vi "Format CSV.vi"(8 "error in (no error)":errorcluster, 9 "delimiter":string=",", 10 "CSV File Input":path, 11 "Original CSV Format":enum16{"Format A", "Format B"}(ring)) -> (0 "error out":errorcluster, 1 "Parcel Length":i32[](array[numeric]), 2 "All Terminal Data":T1(array[cluster]))   [LabVIEW 2017] (continued)
"46:50.6", "46:50.7", "46:50.7", "46:50.7", "46:50.8", "46:50.8", "46:50.8", "46:50.9", "46:50.9", "46:50.9", "46:51.0", "46:51.0", "46:51.0", "46:51.1", "46:51.1", "46:51.1", "46:51.2", "46:51.2", "46:51.2", "46:51.3", "46:51.3", "46:51.3", "46:51.4", "46:51.4", "46:51.4", "46:51.5", "46:51.5", "46:51.5", "46:51.6", "46:51.6", "46:51.6", "46:51.7", "46:51.7", "46:51.7", "46:51.8", "46:51.8", "46:51.8", "46:51.9", "46:51.9", "46:51.9", "46:52.0", "46:52.0", "46:52.0", "46:52.1", "46:52.1", "46:52.1", "46:52.2", "46:52.2", "46:52.2", "46:52.3", "46:52.3", "46:52.3", "46:52.4", "46:52.4", "46:52.4", "46:52.5", "46:52.5", "46:52.5", "46:52.6", "46:52.6", "46:52.6", "46:52.7", "46:52.7", "46:52.7", "46:52.8", "46:52.8", "46:52.8", "46:52.9", "46:52.9", "46:52.9", "46:53.0", "46:53.0", "46:53.0", "46:53.1", "46:53.1", "46:53.1", "46:53.2", "46:53.2", "46:53.2", "46:53.3", "46:53.3", "46:53.3", "46:53.4", "46:53.4", "46:53.4", "46:53.5", "46:53.5", "46:53.5", "46:53.6", "46:53.6", "46:53.6", "46:53.7", "46:53.7", "46:53.7", "46:53.8", "46:53.8", "46:53.8", "46:53.9", "46:53.9", "46:53.9", "46:54.0", "46:54.0", "46:54.0", "46:54.1", "46:54.1", "46:54.1", "46:54.2", "46:54.2", "46:54.2", "46:54.3", "46:54.3", "46:54.3", "46:54.4", "46:54.4", "46:54.4", "46:54.5", "46:54.5", "46:54.5", "46:54.6", "46:54.6", "46:54.6", "46:54.7", "46:54.7", "46:54.7", "46:54.8", "46:54.8", "46:54.8", "46:54.9", "46:54.9", "46:54.9", "46:55.0", "46:55.0", "46:55.0", "46:55.1", "46:55.1", "46:55.1", "46:55.2", "46:55.2", "46:55.2", "46:55.3", "46:55.3", "46:55.3", "46:55.4", "46:55.4", "46:55.4", "46:55.5", "46:55.5", "46:55.5", "46:55.6", "46:55.6", "46:55.6", "46:55.7", "46:55.7", "46:55.7", "46:55.8", "46:55.8", "46:55.8", "46:55.9", "46:55.9", "46:55.9", "46:56.0", "46:56.0", "46:56.0", "46:56.1", "46:56.1", "46:56.1", "46:56.2", "46:56.2", "46:56.2", "46:56.3", "46:56.3", "46:56.3", "46:56.4", "46:56.4", "46:56.4", "46:56.5", "46:56.5", "46:56.5", "46:56.6", "46:56.6", "46:56.6", "46:56.7", "46:56.7", "46:56.7", "46:56.8", "46:56.8", "46:56.8", "46:56.9", "46:56.9", "46:56.9", "46:57.0", "46:57.0", "46:57.0", "46:57.1", "46:57.1", "46:57.1", "46:57.2", "46:57.2", "46:57.2", "46:57.3", "46:57.3", "46:57.3", "46:57.4", "46:57.4", "46:57.4", "46:57.5", "46:57.5", "46:57.5", "46:57.6", "46:57.6", "46:57.6", "46:57.7", "46:57.7", "46:57.7", "46:57.8", "46:57.8", "46:57.8", "46:57.9", "46:57.9", "46:57.9", "46:58.0", "46:58.0", "46:58.0", "46:58.1", "46:58.1", "46:58.1", "46:58.2", "46:58.2", "46:58.2", "46:58.3", "46:58.3", "46:58.3", "46:58.4", "46:58.4", "46:58.4", "46:58.5", "46:58.5", "46:58.5", "46:58.6", "46:58.6", "46:58.6", "46:58.7", "46:58.7", "46:58.7", "46:58.8", "46:58.8", "46:58.8", "46:58.9", "46:58.9", "46:58.9", "46:59.0", "46:59.0", "46:59.0", "46:59.1", "46:59.1", "46:59.1", "46:59.2", "46:59.2", "46:59.2", "46:59.3", "46:59.3", "46:59.3", "46:59.4", "46:59.4", "46:59.4", "46:59.5", "46:59.5", "46:59.5", "46:59.6", "46:59.6", "46:59.6", "46:59.7", "46:59.7", "46:59.7", "46:59.8", "46:59.8", "46:59.8", "46:59.9", "46:59.9", "46:59.9", "47:00.0", "47:00.0", "47:00.0", "47:00.1", "47:00.1", "47:00.1", "47:00.2", "47:00.2", "47:00.2", "47:00.3", "47:00.3", "47:00.3", "47:00.4", "47:00.4", "47:00.4", "47:00.5", "47:00.5", "47:00.5", "47:00.6", "47:00.6", "47:00.6", "47:00.7", "47:00.7", "47:00.7", "47:00.8", "47:00.8", "47:00.8", "47:00.9", "47:00.9", "47:00.9", "47:01.0", "47:01.0", "47:01.0", "47:01.1", "47:01.1", "47:01.1", "47:01.2", "47:01.2", "47:01.2", "47:01.3", "47:01.3", "47:01.3", "47:01.4", "47:01.4", "47:01.4", "47:01.5", "47:01.5", "47:01.5", "47:01.6", "47:01.6", "47:01.6", "47:01.7", "47:01.7", "47:01.7", "47:01.8", "47:01.8", "47:01.8", "47:01.9", "47:01.9", "47:01.9", "47:02.0", "47:02.0", "47:02.0", "47:02.1", "47:02.1", "47:02.1", "47:02.2", "47:02.2", "47:02.2", "47:02.3", "47:02.3", "47:02.3", "47:02.4", "47:02.4", "47:02.4", "47:02.5", "47:02.5", "47:02.5", "47:02.6", "47:02.6", "47:02.6", "47:02.7", "47:02.7", "47:02.7", "47:02.8", "47:02.8", "47:02.8", "47:02.9", "47:02.9", "47:02.9", "47:03.0", "47:03.0", "47:03.0", "47:03.1", "47:03.1", "47:03.1", "47:03.2", "47:03.2", "47:03.2", "47:03.3", "47:03.3", "47:03.3", "47:03.4", "47:03.4", "47:03.4", "47:03.5", "47:03.5", "47:03.5", "47:03.6", "47:03.6", "47:03.6", "47:03.7", "47:03.7", "47:03.7", "47:03.8", "47:03.8", "47:03.8", "47:03.9", "47:03.9", "47:03.9", "47:04.0", "47:04.0", "47:04.0", "47:04.1", "47:04.1", "47:04.1", "47:04.2", "47:04.2", "47:04.2", "47:04.3", "47:04.3", "47:04.3", "47:04.4", "47:04.4", "47:04.4", "47:04.5", "47:04.5", "47:04.5", "47:04.6", "47:04.6", "47:04.6", "47:04.7", "47:04.7", "47:04.7", "47:04.8", "47:04.8", "47:04.8", "47:04.9", "47:04.9", "47:04.9", "47:05.0", "47:05.0", "47:05.0", "47:05.1", "47:05.1", "47:05.1", "47:05.2", "47:05.2", "47:05.2", "47:05.3", "47:05.3", "47:05.3", "47:05.4", "47:05.4", "47:05.4", "47:05.5", "47:05.5", "47:05.5", "47:05.6", "47:05.6", "47:05.6", "47:05.7", "47:05.7", "47:05.7", "47:05.8", "47:05.8", "47:05.8", "47:05.9", "47:05.9", "47:05.9", "47:06.0", "47:06.0", "47:06.0", "47:06.1", "47:06.1", "47:06.1", "47:06.2", "47:06.2", "47:06.2", "47:06.3", "47:06.3", "47:06.3", "47:06.4", "47:06.4", "47:06.4", "47:06.5", "47:06.5", "47:06.5", "47:06.6", "47:06.6", "47:06.6", "47:06.7", "47:06.7", "47:06.7", "47:06.8", "47:06.8", "47:06.8", "47:06.9", "47:06.9", "47:06.9", "47:07.0", "47:07.0", "47:07.0", "47:07.1", "47:07.1", "47:07.1", "47:07.2", "47:07.2", "47:07.2", "47:07.3", "47:07.3", "47:07.3", "47:07.4", "47:07.4", "47:07.4", "47:07.5", "47:07.5", "47:07.5", "47:07.6", "47:07.6", "47:07.6", "47:07.7", "47:07.7", "47:07.7", "47:07.8", "47:07.8", "47:07.8", "47:07.9", "47:07.9", "47:07.9", "47:08.0", "47:08.0", "47:08.0", "47:08.1", "47:08.1", "47:08.1", "47:08.2", "47:08.2", "47:08.2", "47:08.3", "47:08.3", "47:08.3", "47:08.4", "47:08.4", "47:08.4", "47:08.5", "47:08.5", "47:08.5", "47:08.6", "47:08.6", "47:08.6", "47:08.7", "47:08.7", "47:08.7", "47:08.8", "47:08.8", "47:08.8", "47:08.9", "47:08.9", "47:08.9", "47:09.0", "47:09.0", "47:09.0", "47:09.1", "47:09.1", "47:09.1", "47:09.2", "47:09.2", "47:09.2", "47:09.3", "47:09.3", "47:09.3", "47:09.4", "47:09.4", "47:09.4", "47:09.5", "47:09.5", "47:09.5", "47:09.6", "47:09.6", "47:09.6", "47:09.7", "47:09.7", "47:09.7", "47:09.8", "47:09.8", "47:09.8", "47:09.9", "47:09.9", "47:09.9", "47:10.0", "47:10.0", "47:10.0", "47:10.1", "47:10.1", "47:10.1", "47:10.2", "47:10.2", "47:10.2", "47:10.3", "47:10.3", "47:10.3", "47:10.4", "47:10.4", "47:10.4", "47:10.5", "47:10.5", "47:10.5", "47:10.6", "47:10.6", "47:10.6", "47:10.7", "47:10.7", "47:10.7", "47:10.8", "47:10.8", "47:10.8", "47:10.9", "47:10.9", "47:10.9", "47:11.0", "47:11.0", "47:11.0", "47:11.1", "47:11.1", "47:11.1", "47:11.2", "47:11.2", "47:11.2", "47:11.3", "47:11.3", "47:11.3", "47:11.4", "47:11.4", "47:11.4", "47:11.5", "47:11.5", "47:11.5", "47:11.6", "47:11.6", "47:11.6", "47:11.7", "47:11.7", "47:11.7", "47:11.8", "47:11.8", "47:11.8", "47:11.9", "47:11.9", "47:11.9", "47:12.0", "47:12.0", "47:12.0", "47:12.1", "47:12.1", "47:12.1", "47:12.2", "47:12.2", "47:12.2", "47:12.3", "47:12.3", "47:12.3", "47:12.4", "47:12.4", "47:12.4", "47:12.5", "47:12.5", "47:12.5", "47:12.6", "47:12.6", "47:12.6", "47:12.7", "47:12.7", "47:12.7", "47:12.8", "47:12.8", "47:12.8", "47:12.9", "47:12.9", "47:12.9", "47:13.0", "47:13.0", "47:13.0", "47:13.1", "47:13.1", "47:13.1", "47:13.2", "47:13.2", "47:13.2", "47:13.3", "47:13.3", "47:13.3", "47:13.4", "47:13.4", "47:13.4", "47:13.5", "47:13.5", "47:13.5", "47:13.6", "47:13.6", "47:13.6", "47:13.7", "47:13.7", "47:13.7", "47:13.8", "47:13.8", "47:13.8", "47:13.9", "47:13.9", "47:13.9", "47:14.0", "47:14.0", "47:14.0", "47:14.1", "47:14.1", "47:14.1", "47:14.2", "47:14.2", "47:14.2", "47:14.3", "47:14.3", "47:14.3", "47:14.4", "47:14.4", "47:14.4", "47:14.5", "47:14.5", "47:14.5", "47:14.6", "47:14.6", "47:14.6", "47:14.7", "47:14.7", "47:14.7", "47:14.8", "47:14.8", "47:14.8", "47:14.9", "47:14.9", "47:14.9", "47:15.0", "47:15.0", "47:15.0", "47:15.1", "47:15.1", "47:15.1", "47:15.2", "47:15.2", "47:15.2", "47:15.3", "47:15.3", "47:15.3", "47:15.4", "47:15.4", "47:15.4", "47:15.5", "47:15.5", "47:15.5", "47:15.6", "47:15.6", "47:15.6", "47:15.7", "47:15.7", "47:15.7", "47:15.8", "47:15.8", "47:15.8", "47:15.9", "47:15.9", "47:15.9", "47:16.0", "47:16.0", "47:16.0", "47:16.1", "47:16.1", "47:16.1", "47:16.2", "47:16.2", "47:16.2", "47:16.3", "47:16.3", "47:16.3", "47:16.4", "47:16.4", "47:16.4", "47:16.5", "47:16.5", "47:16.5", "47:16.6", "47:16.6", "47:16.6", "47:16.7", "47:16.7", "47:16.7", "47:16.8", "47:16.8", "47:16.8", "47:16.9", "47:16.9", "47:16.9", "47:17.0", "47:17.0", "47:17.0", "47:17.1", "47:17.1", "47:17.1", "47:17.2", "47:17.2", "47:17.2", "47:17.3", "47:17.3", "47:17.3", "47:17.4", "47:17.4", "47:17.4", "47:17.5", "47:17.5", "47:17.5", "47:17.6", "47:17.6", "47:17.6", "47:17.7", "47:17.7", "47:17.7", "47:17.8", "47:17.8", "47:17.8", "47:17.9", "47:17.9", "47:17.9", "47:18.0", "47:18.0", "47:18.0", "47:18.1", "47:18.1", "47:18.1", "47:18.2", "47:18.2", "47:18.2", "47:18.3", "47:18.3", "47:18.3", "47:18.4", "47:18.4", "47:18.4", "47:18.5", "47:18.5", "47:18.5", "47:18.6", "47:18.6", "47:18.6", "47:18.7", "47:18.7", "47:18.7", "47:18.8", "47:18.8", "47:18.8", "47:18.9", "47:18.9", "47:18.9", "47:19.0", "47:19.0", "47:19.0", "47:19.1", "47:19.1", "47:19.1", "47:19.2", "47:19.2", "47:19.2", "47:19.3", "47:19.3", "47:19.3", "47:19.4", "47:19.4", "47:19.4", "47:19.5", "47:19.5", "47:19.5", "47:19.6", "47:19.6", "47:19.6", "47:19.7", "47:19.7", "47:19.7", "47:19.8", "47:19.8", "47:19.8", "47:19.9", "47:19.9", "47:19.9", "47:20.0", "47:20.0", "47:20.0", "47:20.1", "47:20.1", "47:20.1", "47:20.2", "47:20.2", "47:20.2", "47:20.3", "47:20.3", "47:20.3", "47:20.4", "47:20.4", "47:20.4", "47:20.5", "47:20.5", "47:20.5", "47:20.6", "47:20.6", "47:20.6", "47:20.7", "47:20.7", "47:20.7", "47:20.8", "47:20.8", "47:20.8", "47:20.9", "47:20.9", "47:20.9", "47:21.0", "47:21.0", "47:21.0", "47:21.1", "47:21.1", "47:21.1", "47:21.2", "47:21.2", "47:21.2", "47:21.3", "47:21.3", "47:21.3", "47:21.4", "47:21.4", "47:21.4", "47:21.5", "47:21.5", "47:21.5", "47:21.6", "47:21.6", "47:21.6", "47:21.7", "47:21.7", "47:21.7", "47:21.8", "47:21.8", "47:21.8", "47:21.9", "47:21.9", "47:21.9", "47:22.0", "47:22.0", "47:22.0", "47:22.1", "47:22.1", "47:22.1", "47:22.2", "47:22.2", "47:22.2", "47:22.3", "47:22.3", "47:22.3", "47:22.4", "47:22.4", "47:22.4", "47:22.5", "47:22.5", "47:22.5", "47:22.6", "47:22.6", "47:22.6", "47:22.7", "47:22.7", "47:22.7", "47:22.8", "47:22.8", "47:22.8", "47:22.9", "47:22.9", "47:22.9", "47:23.0", "47:23.0", "47:23.0", "47:23.1", "47:23.1", "47:23.1", "47:23.2", "47:23.2", "47:23.2", "47:23.3", "47:23.3", "47:23.3", "47:23.4", "47:23.4", "47:23.4", "47:23.5", "47:23.5", "47:23.5", "47:23.6", "47:23.6", "47:23.6", "47:23.7", "47:23.7", "47:23.7", "47:23.8", "47:23.8", "47:23.8", "47:23.9", "47:23.9", "47:23.9", "47:24.0", "47:24.0", "47:24.0", "47:24.1", "47:24.1", "47:24.1", "47:24.2", "47:24.2", "47:24.2", "47:24.3", "47:24.3", "47:24.3", "47:24.4", "47:24.4", "47:24.4", "47:24.5", "47:24.5", "47:24.5", "47:24.6", "47:24.6", "47:24.6", "47:24.7", "47:24.7", "47:24.7", "47:24.8", "47:24.8", "47:24.8", "47:24.9", "47:24.9", "47:24.9", "47:25.0", "47:25.0", "47:25.0", "47:25.1", "47:25.1", "47:25.1", "47:25.2", "47:25.2", "47:25.2", "47:25.3", "47:25.3", "47:25.3", "47:25.4", "47:25.4", "47:25.4", "47:25.5", "47:25.5", "47:25.5", "47:25.6", "47:25.6", "47:25.6", "47:25.7", "47:25.7", "47:25.7", "47:25.8", "47:25.8", "47:25.8", "47:25.9", "47:25.9", "47:25.9", "47:26.0", "47:26.0", "47:26.0", "47:26.1", "47:26.1", "47:26.1", "47:26.2", "47:26.2", "47:26.2", "47:26.3", "47:26.3", "47:26.3", "47:26.4", "47:26.4", "47:26.4", "47:26.5", "47:26.5", "47:26.5", "47:26.6", "47:26.6", "47:26.6", "47:26.7", "47:26.7", "47:26.7", "47:26.8", "47:26.8", "47:26.8", "47:26.9", "47:26.9", "47:26.9", "47:27.0", "47:27.0", "47:27.0", "47:27.1", "47:27.1", "47:27.1", "47:27.2", "47:27.2", "47:27.2", "47:27.3", "47:27.3", "47:27.3", "47:27.4", "47:27.4", "47:27.4", "47:27.5", "47:27.5", "47:27.5", "47:27.6", "47:27.6", "47:27.6", "47:27.7", "47:27.7", "47:27.7", "47:27.8", "47:27.8", "47:27.8", "47:27.9", "47:27.9", "47:27.9", "47:28.0", "47:28.0", "47:28.0", "47:28.1", "47:28.1", "47:28.1", "47:28.2", "47:28.2", "47:28.2", "47:28.3", "47:28.3", "47:28.3", "47:28.4", "47:28.4", "47:28.4", "47:28.5", "47:28.5", "47:28.5", "47:28.6", "47:28.6", "47:28.6", "47:28.7", "47:28.7", "47:28.7", "47:28.8", "47:28.8", "47:28.8", "47:28.9", "47:28.9", "47:28.9", "47:29.0", "47:29.0", "47:29.0", "47:29.1", "47:29.1", "47:29.1", "47:29.2", "47:29.2", "47:29.2", "47:29.3", "47:29.3", "47:29.3", "47:29.4", "47:29.4", "47:29.4", "47:29.5", "47:29.5", "47:29.5", "47:29.6", "47:29.6", "47:29.6", "47:29.7", "47:29.7", "47:29.7", "47:29.8", "47:29.8", "47:29.8", "47:29.9", "47:29.9", "47:29.9", "47:30.0", "47:30.0", "47:30.0", "47:30.1", "47:30.1", "47:30.1", "47:30.2", "47:30.2", "47:30.2", "47:30.3", "47:30.3", "47:30.3", "47:30.4", "47:30.4", "47:30.4", "47:30.5", "47:30.5", "47:30.5", "47:30.6", "47:30.6", "47:30.6", "47:30.7", "47:30.7", "47:30.7", "47:30.8", "47:30.8", "47:30.8", "47:30.9", "47:30.9", "47:30.9", "47:31.0", "47:31.0", "47:31.0", "47:31.1", "47:31.1", "47:31.1", "47:31.2", "47:31.2", "47:31.2", "47:31.3", "47:31.3", "47:31.3", "47:31.4", "47:31.4", "47:31.4", "47:31.5", "47:31.5", "47:31.5", "47:31.6", "47:31.6", "47:31.6", "47:31.7", "47:31.7", "47:31.7", "47:31.8", "47:31.8", "47:31.8", "47:31.9", "47:31.9", "47:31.9", "47:32.0", "47:32.0", "47:32.0", "47:32.1", "47:32.1", "47:32.1", "47:32.2", "47:32.2", "47:32.2", "47:32.3", "47:32.3", "47:32.3", "47:32.4", "47:32.4", "47:32.4", "47:32.5", "47:32.5", "47:32.5", "47:32.6", "47:32.6", "47:32.6", "47:32.7", "47:32.7", "47:32.7", "47:32.8", "47:32.8", "47:32.8", "47:32.9", "47:32.9", "47:32.9", "47:33.0", "47:33.0", "47:33.0", "47:33.1", "47:33.1", "47:33.1", "47:33.2", "47:33.2", "47:33.2", "47:33.3", "47:33.3", "47:33.3", "47:33.4", "47:33.4", "47:33.4", "47:33.5", "47:33.5", "47:33.5", "47:33.6", "47:33.6", "47:33.6", "47:33.7", "47:33.7", "47:33.7", "47:33.8", "47:33.8", "47:33.8", "47:33.9", "47:33.9", "47:33.9", "47:34.0", "47:34.0", "47:34.0", "47:34.1", "47:34.1", "47:34.1", "47:34.2", "47:34.2", "47:34.2", "47:34.3", "47:34.3", "47:34.3", "47:34.4", "47:34.4", "47:34.4", "47:34.5", "47:34.5", "47:34.5", "47:34.6", "47:34.6", "47:34.6", "47:34.7", "47:34.7", "47:34.7", "47:34.8", "47:34.8", "47:34.8", "47:34.9", "47:34.9", "47:34.9", "47:35.0", "47:35.0", "47:35.0", "47:35.1", "47:35.1", "47:35.1", "47:35.2", "47:35.2", "47:35.2", "47:35.3", "47:35.3", "47:35.3", "47:35.4", "47:35.4", "47:35.4", "47:35.5", "47:35.5", "47:35.5", "47:35.6", "47:35.6", "47:35.6", "47:35.7", "47:35.7", "47:35.7", "47:35.8", "47:35.8", "47:35.8", "47:35.9", "47:35.9", "47:35.9", "47:36.0", "47:36.0", "47:36.0", "47:36.1", "47:36.1", "47:36.1", "47:36.2", "47:36.2", "47:36.2", "47:36.3", "47:36.3", "47:36.3", "47:36.4", "47:36.4", "47:36.4", "47:36.5", "47:36.5", "47:36.5", "47:36.6", "47:36.6", "47:36.6", "47:36.7", "47:36.7", "47:36.7", "47:36.8", "47:36.8", "47:36.8", "47:36.9", "47:36.9", "47:36.9", "47:37.0", "47:37.0", "47:37.0", "47:37.1", "47:37.1", "47:37.1", "47:37.2", "47:37.2", "47:37.2", "47:37.3", "47:37.3", "47:37.3", "47:37.4", "47:37.4", "47:37.4", "47:37.5", "47:37.5", "47:37.5", "47:37.6", "47:37.6", "47:37.6", "47:37.7", "47:37.7", "47:37.7", "47:37.8", "47:37.8", "47:37.8", "47:37.9", "47:37.9", "47:37.9", "47:38.0", "47:38.0", "47:38.0", "47:38.1", "47:38.1", "47:38.1", "47:38.2", "47:38.2", "47:38.2", "47:38.3", "47:38.3", "47:38.3", "47:38.4", "47:38.4", "47:38.4", "47:38.5", "47:38.5", "47:38.5", "47:38.6", "47:38.6", "47:38.6", "47:38.7", "47:38.7", "47:38.7", "47:38.8", "47:38.8", "47:38.8", "47:38.9", "47:38.9", "47:38.9", "47:39.0", "47:39.0", "47:39.0", "47:39.1", "47:39.1", "47:39.1", "47:39.2", "47:39.2", "47:39.2", "47:39.3", "47:39.3", "47:39.3", "47:39.4", "47:39.4", "47:39.4", "47:39.5", "47:39.5", "47:39.5", "47:39.6", "47:39.6", "47:39.6", "47:39.7", "47:39.7", "47:39.7", "47:39.8", "47:39.8", "47:39.8", "47:39.9", "47:39.9", "47:39.9", "47:40.0", "47:40.0", "47:40.0", "47:40.1", "47:40.1", "47:40.1", "47:40.2", "47:40.2", "47:40.2", "47:40.3", "47:40.3", "47:40.3", "47:40.4", "47:40.4", "47:40.4", "47:40.5", "47:40.5", "47:40.5", "47:40.6", "47:40.6", "47:40.6", "47:40.7", "47:40.7", "47:40.7", "47:40.8", "47:40.8", "47:40.8", "47:40.9", "47:40.9", "47:40.9", "47:41.0", "47:41.0", "47:41.0", "47:41.1", "47:41.1", "47:41.1", "47:41.2", "47:41.2", "47:41.2", "47:41.3", "47:41.3", "47:41.3", "47:41.4", "47:41.4", "47:41.4", "47:41.5", "47:41.5", "47:41.5", "47:41.6", "47:41.6", "47:41.6", "47:41.7", "47:41.7", "47:41.7", "47:41.8", "47:41.8", "47:41.8", "47:41.9", "47:41.9", "47:41.9", "47:42.0", "47:42.0", "47:42.0", "47:42.1", "47:42.1", "47:42.1", "47:42.2", "47:42.2", "47:42.2", "47:42.3", "47:42.3", "47:42.3", "47:42.4", "47:42.4", "47:42.4", "47:42.5", "47:42.5", "47:42.5", "47:42.6", "47:42.6", "47:42.6", "47:42.7", "47:42.7", "47:42.7", "47:42.8", "47:42.8", "47:42.8", "47:42.9", "47:42.9", "47:42.9", "47:43.0", "47:43.0", "47:43.0", "47:43.1", "47:43.1", "47:43.1", "47:43.2", "47:43.2", "47:43.2", "47:43.3", "47:43.3", "47:43.3", "47:43.4", "47:43.4", "47:43.4", "47:43.5", "47:43.5", "47:43.5", "47:43.6", "47:43.6", "47:43.6", "47:43.7", "47:43.7", "47:43.7", "47:43.8", "47:43.8", "47:43.8", "47:43.9", "47:43.9", "47:43.9", "47:44.0", "47:44.0", "47:44.0", "47:44.1", "47:44.1", "47:44.1", "47:44.2", "47:44.2", "47:44.2", "47:44.3", "47:44.3", "47:44.3", "47:44.4", "47:44.4", "47:44.4", "47:44.5", "47:44.5", "47:44.5", "47:44.6", "47:44.6", "47:44.6", "47:44.7", "47:44.7", "47:44.7", "47:44.8", "47:44.8", "47:44.8", "47:44.9", "47:44.9", "47:44.9", "47:45.0", "47:45.0", "47:45.0", "47:45.1", "47:45.1", "47:45.1", "47:45.2", "47:45.2", "47:45.2", "47:45.3", "47:45.3", "47:45.3", "47:45.4", "47:45.4", "47:45.4", "47:45.5", "47:45.5", "47:45.5", "47:45.6", "47:45.6", "47:45.6", "47:45.7", "47:45.7", "47:45.7", "47:45.8", "47:45.8", "47:45.8", "47:45.9", "47:45.9", "47:45.9", "47:46.0", "47:46.0", "47:46.0", "47:46.1", "47:46.1", "47:46.1", "47:46.2", "47:46.2", "47:46.2", "47:46.3", "47:46.3", "47:46.3", "47:46.4", "47:46.4", "47:46.4", "47:46.5", "47:46.5", "47:46.5", "47:46.6", "47:46.6", "47:46.6", "47:46.7", "47:46.7", "47:46.7", "47:46.8", "47:46.8", "47:46.8", "47:46.9", "47:46.9", "47:46.9", "47:47.0", "47:47.0", "47:47.0", "47:47.1", "47:47.1", "47:47.1", "47:47.2", "47:47.2", "47:47.2", "47:47.3", "47:47.3", "47:47.3", "47:47.4", "47:47.4", "47:47.4", "47:47.5", "47:47.5", "47:47.5", "47:47.6", "47:47.6", "47:47.6", "47:47.7", "47:47.7", "47:47.7", "47:47.8", "47:47.8", "47:47.8", "47:47.9", "47:47.9", "47:47.9", "47:48.0", "47:48.0", "47:48.0", "47:48.1", "47:48.1", "47:48.1", "47:48.2", "47:48.2", "47:48.2", "47:48.3", "47:48.3", "47:48.3", "47:48.4", "47:48.4", "47:48.4", "47:48.5", "47:48.5", "47:48.5", "47:48.6", "47:48.6", "47:48.6", "47:48.7", "47:48.7", "47:48.7", "47:48.8", "47:48.8", "47:48.8", "47:48.9", "47:48.9", "47:48.9", "47:49.0", "47:49.0", "47:49.0", "47:49.1", "47:49.1", "47:49.1", "47:49.2", "47:49.2", "47:49.2", "47:49.3", "47:49.3", "47:49.3", "47:49.4", "47:49.4", "47:49.4", "47:49.5", "47:49.5", "47:49.5", "47:49.6", "47:49.6", "47:49.6", "47:49.7", "47:49.7", "47:49.7", "47:49.8", "47:49.8", "47:49.8", "47:49.9", "47:49.9", "47:49.9", "47:50.0", "47:50.0", "47:50.0", "47:50.1", "47:50.1", "47:50.1", "47:50.2", "47:50.2", "47:50.2", "47:50.3", "47:50.3", "47:50.3", "47:50.4", "47:50.4", "47:50.4", "47:50.5", "47:50.5", "47:50.5", "47:50.6", "47:50.6", "47:50.6", "47:50.7", "47:50.7", "47:50.7", "47:50.8", "47:50.8", "47:50.8", "47:50.9", "47:50.9", "47:50.9", "47:51.0", "47:51.0", "47:51.0", "47:51.1", "47:51.1", "47:51.1", "47:51.2", "47:51.2", "47:51.2", "47:51.3", "47:51.3", "47:51.3", "47:51.4", "47:51.4", "47:51.4", "47:51.5", "47:51.5", "47:51.5", "47:51.6", "47:51.6", "47:51.6", "47:51.7", "47:51.7", "47:51.7", "47:51.8", "47:51.8", "47:51.8", "47:51.9", "47:51.9", "47:51.9", "47:52.0", "47:52.0", "47:52.0", "47:52.1", "47:52.1", "47:52.1", "47:52.2", "47:52.2", "47:52.2", "47:52.3", "47:52.3", "47:52.3", "47:52.4", "47:52.4", "47:52.4", "47:52.5", "47:52.5", "47:52.5", "47:52.6", "47:52.6", "47:52.6", "47:52.7", "47:52.7", "47:52.7", "47:52.8", "47:52.8", "47:52.8", "47:52.9", "47:52.9", "47:52.9", "47:53.0", "47:53.0", "47:53.0", "47:53.1", "47:53.1", "47:53.1", "47:53.2", "47:53.2", "47:53.2", "47:53.3", "47:53.3", "47:53.3", "47:53.4", "47:53.4", "47:53.4", "47:53.5", "47:53.5", "47:53.5", "47:53.6", "47:53.6", "47:53.6", "47:53.7", "47:53.7", "47:53.7", "47:53.8", "47:53.8", "47:53.8", "47:53.9", "47:53.9", "47:53.9", "47:54.0", "47:54.0", "47:54.0", "47:54.1", "47:54.1", "47:54.1", "47:54.2", "47:54.2", "47:54.2", "47:54.3", "47:54.3", "47:54.3", "47:54.4", "47:54.4", "47:54.4", "47:54.5", "47:54.5", "47:54.5", "47:54.6", "47:54.6", "47:54.6", "47:54.7", "47:54.7", "47:54.7", "47:54.8", "47:54.8", "47:54.8", "47:54.9", "47:54.9", "47:54.9", "47:55.0", "47:55.0", "47:55.0", "47:55.1", "47:55.1", "47:55.1", "47:55.2", "47:55.2", "47:55.2", "47:55.3", "47:55.3", "47:55.3", "47:55.4", "47:55.4", "47:55.4", "47:55.5", "47:55.5", "47:55.5", "47:55.6", "47:55.6", "47:55.6", "47:55.7", "47:55.7", "47:55.7", "47:55.8", "47:55.8", "47:55.8", "47:55.9", "47:55.9", "47:55.9", "47:56.0", "47:56.0", "47:56.0", "47:56.1", "47:56.1", "47:56.1", "47:56.2", "47:56.2", "47:56.2", "47:56.3", "47:56.3", "47:56.3", "47:56.4", "47:56.4", "47:56.4", "47:56.5", "47:56.5", "47:56.5", "47:56.6", "47:56.6", "47:56.6", "47:56.7", "47:56.7", "47:56.7", "47:56.8", "47:56.8", "47:56.8", "47:56.9", "47:56.9", "47:56.9", "47:57.0", "47:57.0", "47:57.0", "47:57.1", "47:57.1", "47:57.1", "47:57.2", "47:57.2", "47:57.2", "47:57.3", "47:57.3", "47:57.3", "47:57.4", "47:57.4", "47:57.4", "47:57.5", "47:57.5", "47:57.5", "47:57.6", "47:57.6", "47:57.6", "47:57.7", "47:57.7", "47:57.7", "47:57.8", "47:57.8", "47:57.8", "47:57.9", "47:57.9", "47:57.9", "47:58.0", "47:58.0", "47:58.0", "47:58.1", "47:58.1", "47:58.1", "47:58.2", "47:58.2", "47:58.2", "47:58.3", "47:58.3", "47:58.3", "47:58.4", "47:58.4", "47:58.4", "47:58.5", "47:58.5", "47:58.5", "47:58.6", "47:58.6", "47:58.6", "47:58.7", "47:58.7", "47:58.7", "47:58.8", "47:58.8", "47:58.8", "47:58.9", "47:58.9", "47:58.9", "47:59.0", "47:59.0", "47:59.0", "47:59.1", "47:59.1", "47:59.1", "47:59.2", "47:59.2", "47:59.2", "47:59.3", "47:59.3", "47:59.3", "47:59.4", "47:59.4", "47:59.4", "47:59.5", "47:59.5", "47:59.5", "47:59.6", "47:59.6", "47:59.6", "47:59.7", "47:59.7", "47:59.7", "47:59.8", "47:59.8", "47:59.8", "47:59.9", "47:59.9", "47:59.9", "48:00.0", "48:00.0", "48:00.0", "48:00.1", "48:00.1", "48:00.1", "48:00.2", "48:00.2", "48:00.2", "48:00.3", "48:00.3", "48:00.3", "48:00.4", "48:00.4", "48:00.4", "48:00.5", "48:00.5", "48:00.5", "48:00.6", "48:00.6", "48:00.6", "48:00.7", "48:00.7", "48:00.7", "48:00.8", "48:00.8", "48:00.8", "48:00.9", "48:00.9", "48:00.9", "48:01.0", "48:01.0", "48:01.0", "48:01.1", "48:01.1", "48:01.1", "48:01.2", "48:01.2", "48:01.2", "48:01.3", "48:01.3", "48:01.3", "48:01.4", "48:01.4", "48:01.4", "48:01.5", "48:01.5", "48:01.5", "48:01.6", "48:01.6", "48:01.6", "48:01.7", "48:01.7", "48:01.7", "48:01.8", "48:01.8", "48:01.8", "48:01.9", "48:01.9", "48:01.9", "48:02.0", "48:02.0", "48:02.0", "48:02.1", "48:02.1", "48:02.1", "48:02.2", "48:02.2", "48:02.2", "48:02.3", "48:02.3", "48:02.3", "48:02.4", "48:02.4", "48:02.4", "48:02.5", "48:02.5", "48:02.5", "48:02.6", "48:02.6", "48:02.6", "48:02.7", "48:02.7", "48:02.7", "48:02.8", "48:02.8", "48:02.8", "48:02.9", "48:02.9", "48:02.9", "48:03.0", "48:03.0", "48:03.0", "48:03.1", "48:03.1", "48:03.1", "48:03.2", "48:03.2", "48:03.2", "48:03.3", "48:03.3", "48:03.3", "48:03.4", "48:03.4", "48:03.4", "48:03.5", "48:03.5", "48:03.5", "48:03.6", "48:03.6", "48:03.6", "48:03.7", "48:03.7", "48:03.7", "48:03.8", "48:03.8", "48:03.8", "48:03.9", "48:03.9", "48:03.9", "48:04.0", "48:04.0", "48:04.0", "48:04.1", "48:04.1", "48:04.1", "48:04.2", "48:04.2", "48:04.2", "48:04.3", "48:04.3", "48:04.3", "48:04.4", "48:04.4", "48:04.4", "48:04.5", "48:04.5", "48:04.5", "48:04.6", "48:04.6", "48:04.6", "48:04.7", "48:04.7", "48:04.7", "48:04.8", "48:04.8", "48:04.8", "48:04.9", "48:04.9", "48:04.9", "48:05.0", "48:05.0", "48:05.0", "48:05.1", "48:05.1", "48:05.1", "48:05.2", "48:05.2", "48:05.2", "48:05.3", "48:05.3", "48:05.3", "48:05.4", "48:05.4", "48:05.4", "48:05.5", "48:05.5", "48:05.5", "48:05.6", "48:05.6", "48:05.6", "48:05.7", "48:05.7", "48:05.7", "48:05.8", "48:05.8", "48:05.8", "48:05.9", "48:05.9", "48:05.9", "48:06.0", "48:06.0", "48:06.0", "48:06.1", "48:06.1", "48:06.1", "48:06.2", "48:06.2", "48:06.2", "48:06.3", "48:06.3", "48:06.3", "48:06.4", "48:06.4", "48:06.4", "48:06.5", "48:06.5", "48:06.5", "48:06.6", "48:06.6", "48:06.6", "48:06.7", "48:06.7", "48:06.7", "48:06.8", "48:06.8", "48:06.8", "48:06.9", "48:06.9", "48:06.9", "48:07.0", "48:07.0", "48:07.0", "48:07.1", "48:07.1", "48:07.1", "48:07.2", "48:07.2", "48:07.2", "48:07.3", "48:07.3", "48:07.3", "48:07.4", "48:07.4", "48:07.4", "48:07.5", "48:07.5", "48:07.5", "48:07.6", "48:07.6", "48:07.6", "48:07.7", "48:07.7", "48:07.7", "48:07.8", "48:07.8", "48:07.8", "48:07.9", "48:07.9", "48:07.9", "48:08.0", "48:08.0", "48:08.0", "48:08.1", "48:08.1", "48:08.1", "48:08.2", "48:08.2", "48:08.2", "48:08.3", "48:08.3", "48:08.3", "48:08.4", "48:08.4", "48:08.4", "48:08.5", "48:08.5", "48:08.5", "48:08.6", "48:08.6", "48:08.6", "48:08.7", "48:08.7", "48:08.7", "48:08.8", "48:08.8", "48:08.8", "48:08.9", "48:08.9", "48:08.9", "48:09.0", "48:09.0", "48:09.0", "48:09.1", "48:09.1", "48:09.1", "48:09.2", "48:09.2", "48:09.2", "48:09.3", "48:09.3", "48:09.3", "48:09.4", "48:09.4", "48:09.4", "48:09.5", "48:09.5", "48:09.5", "48:09.6", "48:09.6", "48:09.6", "48:09.7", "48:09.7", "48:09.7", "48:09.8", "48:09.8", "48:09.8", "48:09.9", "48:09.9", "48:09.9", "48:10.0", "48:10.0", "48:10.0", "48:10.1", "48:10.1", "48:10.1", "48:10.2", "48:10.2", "48:10.2", "48:10.3", "48:10.3", "48:10.3", "48:10.4", "48:10.4", "48:10.4", "48:10.5", "48:10.5", "48:10.5", "48:10.6", "48:10.6", "48:10.6", "48:10.7", "48:10.7", "48:10.7", "48:10.8", "48:10.8", "48:10.8", "48:10.9", "48:10.9", "48:10.9", "48:11.0", "48:11.0", "48:11.0", "48:11.1", "48:11.1", "48:11.1", "48:11.2", "48:11.2", "48:11.2", "48:11.3", "48:11.3", "48:11.3", "48:11.4", "48:11.4", "48:11.4", "48:11.5", "48:11.5", "48:11.5", "48:11.6", "48:11.6", "48:11.6", "48:11.7", "48:11.7", "48:11.7", "48:11.8", "48:11.8", "48:11.8", "48:11.9", "48:11.9", "48:11.9", "48:12.0", "48:12.0", "48:12.0", "48:12.1", "48:12.1", "48:12.1", "48:12.2", "48:12.2", "48:12.2", "48:12.3", "48:12.3", "48:12.3", "48:12.4", "48:12.4", "48:12.4", "48:12.5", "48:12.5", "48:12.5", "48:12.6", "48:12.6", "48:12.6", "48:12.7", "48:12.7", "48:12.7", "48:12.8", "48:12.8", "48:12.8", "48:12.9", "48:12.9", "48:12.9", "48:13.0", "48:13.0", "48:13.0", "48:13.1", "48:13.1", "48:13.1", "48:13.2", "48:13.2", "48:13.2", "48:13.3", "48:13.3", "48:13.3", "48:13.4", "48:13.4", "48:13.4", "48:13.5", "48:13.5", "48:13.5", "48:13.6", "48:13.6", "48:13.6", "48:13.7", "48:13.7", "48:13.7", "48:13.8", "48:13.8", "48:13.8", "48:13.9", "48:13.9", "48:13.9", "48:14.0", "48:14.0", "48:14.0", "48:14.1", "48:14.1", "48:14.1", "48:14.2", "48:14.2", "48:14.2", "48:14.3", "48:14.3", "48:14.3", "48:14.4", "48:14.4", "48:14.4", "48:14.5", "48:14.5", "48:14.5", "48:14.6", "48:14.6", "48:14.6", "48:14.7", "48:14.7", "48:14.7", "48:14.8", "48:14.8", "48:14.8", "48:14.9", "48:14.9", "48:14.9", "48:15.0", "48:15.0", "48:15.0", "48:15.1", "48:15.1", "48:15.1", "48:15.2", "48:15.2", "48:15.2", "48:15.3", "48:15.3", "48:15.3", "48:15.4", "48:15.4", "48:15.4", "48:15.5", "48:15.5", "48:15.5", "48:15.6", "48:15.6", "48:15.6", "48:15.7", "48:15.7", "48:15.7", "48:15.8", "48:15.8", "48:15.8", "48:15.9", "48:15.9", "48:15.9", "48:16.0", "48:16.0", "48:16.0", "48:16.1", "48:16.1", "48:16.1", "48:16.2", "48:16.2", "48:16.2", "48:16.3", "48:16.3", "48:16.3", "48:16.4", "48:16.4", "48:16.4", "48:16.5", "48:16.5", "48:16.5", "48:16.6", "48:16.6", "48:16.6", "48:16.7", "48:16.7", "48:16.7", "48:16.8", "48:16.8", "48:16.8", "48:16.9", "48:16.9", "48:16.9", "48:17.0", "48:17.0", "48:17.0", "48:17.1", "48:17.1", "48:17.1", "48:17.2", "48:17.2", "48:17.2", "48:17.3", "48:17.3", "48:17.3", "48:17.4", "48:17.4", "48:17.4", "48:17.5", "48:17.5", "48:17.5", "48:17.6", "48:17.6", "48:17.6", "48:17.7", "48:17.7", "48:17.7", "48:17.8", "48:17.8", "48:17.8", "48:17.9", "48:17.9", "48:17.9", "48:18.0", "48:18.0", "48:18.0", "48:18.1", "48:18.1", "48:18.1", "48:18.2", "48:18.2", "48:18.2", "48:18.3", "48:18.3", "48:18.3", "48:18.4", "48:18.4", "48:18.4", "48:18.5", "48:18.5", "48:18.5", "48:18.6", "48:18.6", "48:18.6", "48:18.7", "48:18.7", "48:18.7", "48:18.8", "48:18.8", "48:18.8", "48:18.9", "48:18.9", "48:18.9", "48:19.0", "48:19.0", "48:19.0", "48:19.1", "48:19.1", "48:19.1", "48:19.2", "48:19.2", "48:19.2", "48:19.3", "48:19.3", "48:19.3", "48:19.4", "48:19.4", "48:19.4", "48:19.5", "48:19.5", "48:19.5", "48:19.6", "48:19.6", "48:19.6", "48:19.7", "48:19.7", "48:19.7", "48:19.8", "48:19.8", "48:19.8", "48:19.9", "48:19.9", "48:19.9", "48:20.0", "48:20.0", "48:20.0", "48:20.1", "48:20.1", "48:20.1", "48:20.2", "48:20.2", "48:20.2", "48:20.3", "48:20.3", "48:20.3", "48:20.4", "48:20.4", "48:20.4", "48:20.5", "48:20.5", "48:20.5", "48:20.6", "48:20.6", "48:20.6", "48:20.7", "48:20.7", "48:20.7", "48:20.8", "48:20.8", "48:20.8", "48:20.9", "48:20.9", "48:20.9", "48:21.0", "48:21.0", "48:21.0", "48:21.1", "48:21.1", "48:21.1", "48:21.2", "48:21.2", "48:21.2", "48:21.3", "48:21.3", "48:21.3", "48:21.4", "48:21.4", "48:21.4", "48:21.5", "48:21.5", "48:21.5", "48:21.6", "48:21.6", "48:21.6", "48:21.7", "48:21.7", "48:21.7", "48:21.8", "48:21.8", "48:21.8", "48:21.9", "48:21.9", "48:21.9", "48:22.0", "48:22.0", "48:22.0", "48:22.1", "48:22.1", "48:22.1", "48:22.2", "48:22.2", "48:22.2", "48:22.3", "48:22.3", "48:22.3", "48:22.4", "48:22.4", "48:22.4", "48:22.5", "48:22.5", "48:22.5", "48:22.6", "48:22.6", "48:22.6", "48:22.7", "48:22.7", "48:22.7", "48:22.8", "48:22.8", "48:22.8", "48:22.9", "48:22.9", "48:22.9", "48:23.0", "48:23.0", "48:23.0", "48:23.1", "48:23.1", "48:23.1", "48:23.2", "48:23.2", "48:23.2", "48:23.3", "48:23.3", "48:23.3", "48:23.4", "48:23.4", "48:23.4", "48:23.5", "48:23.5", "48:23.5", "48:23.6", "48:23.6", "48:23.6", "48:23.7", "48:23.7", "48:23.7", "48:23.8", "48:23.8", "48:23.8", "48:23.9", "48:23.9", "48:23.9", "48:24.0", "48:24.0", "48:24.0", "48:24.1", "48:24.1", "48:24.1", "48:24.2", "48:24.2", "48:24.2", "48:24.3", "48:24.3", "48:24.3", "48:24.4", "48:24.4", "48:24.4", "48:24.5", "48:24.5", "48:24.5", "48:24.6", "48:24.6", "48:24.6", "48:24.7", "48:24.7", "48:24.7", "48:24.8", "48:24.8", "48:24.8", "48:24.9", "48:24.9", "48:24.9", "48:25.0", "48:25.0", "48:25.0", "48:25.1", "48:25.1", "48:25.1", "48:25.2", "48:25.2", "48:25.2", "48:25.3", "48:25.3", "48:25.3", "48:25.4", "48:25.4", "48:25.4", "48:25.5", "48:25.5", "48:25.5", "48:25.6", "48:25.6", "48:25.6", "48:25.7", "48:25.7", "48:25.7", "48:25.8", "48:25.8", "48:25.8", "48:25.9", "48:25.9", "48:25.9", "48:26.0", "48:26.0", "48:26.0", "48:26.1", "48:26.1", "48:26.1", "48:26.2", "48:26.2", "48:26.2", "48:26.3", "48:26.3", "48:26.3", "48:26.4", "48:26.4", "48:26.4", "48:26.5", "48:26.5", "48:26.5", "48:26.6", "48:26.6", "48:26.6", "48:26.7", "48:26.7", "48:26.7", "48:26.8", "48:26.8", "48:26.8", "48:26.9", "48:26.9", "48:26.9", "48:27.0", "48:27.0", "48:27.0", "48:27.1", "48:27.1", "48:27.1", "48:27.2", "48:27.2", "48:27.2", "48:27.3", "48:27.3", "48:27.3", "48:27.4", "48:27.4", "48:27.4", "48:27.5", "48:27.5", "48:27.5", "48:27.6", "48:27.6", "48:27.6", "48:27.7", "48:27.7", "48:27.7", "48:27.8", "48:27.8", "48:27.8", "48:27.9", "48:27.9", "48:27.9", "48:28.0", "48:28.0", "48:28.0", "48:28.1", "48:28.1", "48:28.1", "48:28.2", "48:28.2", "48:28.2", "48:28.3", "48:28.3", "48:28.3", "48:28.4", "48:28.4", "48:28.4", "48:28.5", "48:28.5", "48:28.5", "48:28.6", "48:28.6", "48:28.6", "48:28.7", "48:28.7", "48:28.7", "48:28.8", "48:28.8", "48:28.8", "48:28.9", "48:28.9", "48:28.9", "48:29.0", "48:29.0", "48:29.0", "48:29.1", "48:29.1", "48:29.1", "48:29.2", "48:29.2", "48:29.2", "48:29.3", "48:29.3", "48:29.3", "48:29.4", "48:29.4", "48:29.4", "48:29.5", "48:29.5", "48:29.5", "48:29.6", "48:29.6", "48:29.6", "48:29.7", "48:29.7", "48:29.7", "48:29.8", "48:29.8", "48:29.8", "48:29.9", "48:29.9", "48:29.9", "48:30.0", "48:30.0", "48:30.0", "48:30.1", "48:30.1", "48:30.1", "48:30.2", "48:30.2", "48:30.2", "48:30.3", "48:30.3", "48:30.3", "48:30.4", "48:30.4", "48:30.4", "48:30.5", "48:30.5", "48:30.5", "48:30.6", "48:30.6", "48:30.6", "48:30.7", "48:30.7", "48:30.7", "48:30.8", "48:30.8", "48:30.8", "48:30.9", "48:30.9", "48:30.9", "48:31.0", "48:31.0", "48:31.0", "48:31.1", "48:31.1", "48:31.1", "48:31.2", "48:31.2", "48:31.2", "48:31.3", "48:31.3", "48:31.3", "48:31.4", "48:31.4", "48:31.4", "48:31.5", "48:31.5", "48:31.5", "48:31.6", "48:31.6", "48:31.6", "48:31.7", "48:31.7", "48:31.7", "48:31.8", "48:31.8", "48:31.8", "48:31.9", "48:31.9", "48:31.9", "48:32.0", "48:32.0", "48:32.0", "48:32.1", "48:32.1", "48:32.1", "48:32.2", "48:32.2", "48:32.2", "48:32.3", "48:32.3", "48:32.3", "48:32.4", "48:32.4", "48:32.4", "48:32.5", "48:32.5", "48:32.5", "48:32.6", "48:32.6", "48:32.6", "48:32.7", "48:32.7", "48:32.7", "48:32.8", "48:32.8", "48:32.8", "48:32.9", "48:32.9", "48:32.9", "48:33.0", "48:33.0", "48:33.0", "48:33.1", "48:33.1", "48:33.1", "48:33.2", "48:33.2", "48:33.2", "48:33.3", "48:33.3", "48:33.3", "48:33.4", "48:33.4", "48:33.4", "48:33.5", "48:33.5", "48:33.5", "48:33.6", "48:33.6", "48:33.6", "48:33.7", "48:33.7", "48:33.7", "48:33.8", "48:33.8", "48:33.8", "48:33.9", "48:33.9", "48:33.9", "48:34.0", "48:34.0", "48:34.0", "48:34.1", "48:34.1", "48:34.1", "48:34.2", "48:34.2", "48:34.2", "48:34.3", "48:34.3", "48:34.3", "48:34.4", "48:34.4", "48:34.4", "48:34.5", "48:34.5", "48:34.5", "48:34.6", "48:34.6", "48:34.6", "48:34.7", "48:34.7", "48:34.7", "48:34.8", "48:34.8", "48:34.8", "48:34.9", "48:34.9", "48:34.9", "48:35.0", "48:35.0", "48:35.0", "48:35.1", "48:35.1", "48:35.1", "48:35.2", "48:35.2", "48:35.2", "48:35.3", "48:35.3", "48:35.3", "48:35.4", "48:35.4", "48:35.4", "48:35.5", "48:35.5", "48:35.5", "48:35.6", "48:35.6", "48:35.6", "48:35.7", "48:35.7", "48:35.7", "48:35.8", "48:35.8", "48:35.8", "48:35.9", "48:35.9", "48:35.9", "48:36.0", "48:36.0", "48:36.0", "48:36.1", "48:36.1", "48:36.1", "48:36.2", "48:36.2", "48:36.2", "48:36.3", "48:36.3", "48:36.3", "48:36.4", "48:36.4", "48:36.4", "48:36.5", "48:36.5", "48:36.5", "48:36.6", "48:36.6", "48:36.6", "48:36.7", "48:36.7", "48:36.7", "48:36.8", "48:36.8", "48:36.8", "48:36.9", "48:36.9", "48:36.9", "48:37.0", "48:37.0", "48:37.0", "48:37.1", "48:37.1", "48:37.1", "48:37.2", "48:37.2", "48:37.2", "48:37.3", "48:37.3", "48:37.3", "48:37.4", "48:37.4", "48:37.4", "48:37.5", "48:37.5", "48:37.5", "48:37.6", "48:37.6", "48:37.6", "48:37.7", "48:37.7", "48:37.7", "48:37.8", "48:37.8", "48:37.8", "48:37.9", "48:37.9", "48:37.9", "48:38.0", "48:38.0", "48:38.0", "48:38.1", "48:38.1", "48:38.1", "48:38.2", "48:38.2", "48:38.2", "48:38.3", "48:38.3", "48:38.3", "48:38.4", "48:38.4", "48:38.4", "48:38.5", "48:38.5", "48:38.5", "48:38.6", "48:38.6", "48:38.6", "48:38.7", "48:38.7", "48:38.7", "48:38.8", "48:38.8", "48:38.8", "48:38.9", "48:38.9", "48:38.9", "48:39.0", "48:39.0", "48:39.0", "48:39.1", "48:39.1", "48:39.1", "48:39.2", "48:39.2", "48:39.2", "48:39.3", "48:39.3", "48:39.3", "48:39.4", "48:39.4", "48:39.4", "48:39.5", "48:39.5", "48:39.5", "48:39.6", "48:39.6", "48:39.6", "48:39.7", "48:39.7", "48:39.7", "48:39.8", "48:39.8", "48:39.8", "48:39.9", "48:39.9", "48:39.9", "48:40.0", "48:40.0", "48:40.0", "48:40.1", "48:40.1", "48:40.1", "48:40.2", "48:40.2", "48:40.2", "48:40.3", "48:40.3", "48:40.3", "48:40.4", "48:40.4", "48:40.4", "48:40.5", "48:40.5", "48:40.5", "48:40.6", "48:40.6", "48:40.6", "48:40.7", "48:40.7", "48:40.7", "48:40.8", "48:40.8", "48:40.8", "48:40.9", "48:40.9", "48:40.9", "48:41.0", "48:41.0", "48:41.0", "48:41.1", "48:41.1", "48:41.1", "48:41.2", "48:41.2", "48:41.2", "48:41.3", "48:41.3", "48:41.3", "48:41.4", "48:41.4", "48:41.4", "48:41.5", "48:41.5", "48:41.5", "48:41.6", "48:41.6", "48:41.6", "48:41.7", "48:41.7", "48:41.7", "48:41.8", "48:41.8", "48:41.8", "48:41.9", "48:41.9", "48:41.9", "48:42.0", "48:42.0", "48:42.0", "48:42.1", "48:42.1", "48:42.1", "48:42.2", "48:42.2", "48:42.2", "48:42.3", "48:42.3", "48:42.3", "48:42.4", "48:42.4", "48:42.4", "48:42.5", "48:42.5", "48:42.5", "48:42.6", "48:42.6", "48:42.6", "48:42.7", "48:42.7", "48:42.7", "48:42.8", "48:42.8", "48:42.8", "48:42.9", "48:42.9", "48:42.9", "48:43.0", "48:43.0", "48:43.0", "48:43.1", "48:43.1", "48:43.1", "48:43.2", "48:43.2", "48:43.2", "48:43.3", "48:43.3", "48:43.3", "48:43.4", "48:43.4", "48:43.4", "48:43.5", "48:43.5", "48:43.5", "48:43.6", "48:43.6", "48:43.6", "48:43.7", "48:43.7", "48:43.7", "48:43.8", "48:43.8", "48:43.8", "48:43.9", "48:43.9", "48:43.9", "48:44.0", "48:44.0", "48:44.0", "48:44.1", "48:44.1", "48:44.1", "48:44.2", "48:44.2", "48:44.2", "48:44.3", "48:44.3", "48:44.3", "48:44.4", "48:44.4", "48:44.4", "48:44.5", "48:44.5", "48:44.5", "48:44.6", "48:44.6", "48:44.6", "48:44.7", "48:44.7", "48:44.7", "48:44.8", "48:44.8", "48:44.8", "48:44.9", "48:44.9", "48:44.9", "48:45.0", "48:45.0", "48:45.0", "48:45.1", "48:45.1", "48:45.1", "48:45.2", "48:45.2", "48:45.2", "48:45.3", "48:45.3", "48:45.3", "48:45.4", "48:45.4", "48:45.4", "48:45.5", "48:45.5", "48:45.5", "48:45.6", "48:45.6", "48:45.6", "48:45.7", "48:45.7", "48:45.7", "48:45.8", "48:45.8", "48:45.8", "48:45.9", "48:45.9", "48:45.9", "48:46.0", "48:46.0", "48:46.0", "48:46.1", "48:46.1", "48:46.1", "48:46.2", "48:46.2", "48:46.2", "48:46.3", "48:46.3", "48:46.3", "48:46.4", "48:46.4", "48:46.4", "48:46.5", "48:46.5", "48:46.5", "48:46.6", "48:46.6", "48:46.6", "48:46.7", "48:46.7", "48:46.7", "48:46.8", "48:46.8", "48:46.8", "48:46.9", "48:46.9", "48:46.9", "48:47.0", "48:47.0", "48:47.0", "48:47.1", "48:47.1", "48:47.1", "48:47.2", "48:47.2", "48:47.2", "48:47.3", "48:47.3", "48:47.3", "48:47.4", "48:47.4", "48:47.4", "48:47.5", "48:47.5", "48:47.5", "48:47.6", "48:47.6", "48:47.6", "48:47.7", "48:47.7", "48:47.7", "48:47.8", "48:47.8", "48:47.8", "48:47.9", "48:47.9", "48:47.9", "48:48.0", "48:48.0", "48:48.0", "48:48.1", "48:48.1", "48:48.1", "48:48.2", "48:48.2", "48:48.2", "48:48.3", "48:48.3", "48:48.3", "48:48.4", "48:48.4", "48:48.4", "48:48.5", "48:48.5", "48:48.5", "48:48.6", "48:48.6", "48:48.6", "48:48.7", "48:48.7", "48:48.7", "48:48.8", "48:48.8", "48:48.8", "48:48.9", "48:48.9", "48:48.9", "48:49.0", "48:49.0", "48:49.0", "48:49.1", "48:49.1", "48:49.1", "48:49.2", "48:49.2", "48:49.2", "48:49.3", "48:49.3", "48:49.3", "48:49.4", "48:49.4", "48:49.4", "48:49.5", "48:49.5", "48:49.5", "48:49.6", "48:49.6", "48:49.6", "48:49.7", "48:49.7", "48:49.7", "48:49.8", "48:49.8", "48:49.8", "48:49.9", "48:49.9", "48:49.9", "48:50.0", "48:50.0", "48:50.0", "48:50.1", "48:50.1", "48:50.1", "48:50.2", "48:50.2", "48:50.2", "48:50.3", "48:50.3", "48:50.3", "48:50.4", "48:50.4", "48:50.4", "48:50.5", "48:50.5", "48:50.5", "48:50.6", "48:50.6", "48:50.6", "48:50.7", "48:50.7", "48:50.7", "48:50.8", "48:50.8", "48:50.8", "48:50.9", "48:50.9", "48:50.9", "48:51.0", "48:51.0", "48:51.0", "48:51.1", "48:51.1", "48:51.1", "48:51.2", "48:51.2", "48:51.2", "48:51.3", "48:51.3", "48:51.3", "48:51.4", "48:51.4", "48:51.4", "48:51.5", "48:51.5", "48:51.5", "48:51.6", "48:51.6", "48:51.6", "48:51.7", "48:51.7", "48:51.7", "48:51.8", "48:51.8",
